vi "WS_BackCheck_Serial.vi"(2 "stationName":string, 3 "serialNumber":string) -> (0 "ProcessName":string, 1 "Status":i8)   [LabVIEW 2022 SP3]
uses:
  C:/Users/K90011729/OneDrive - Kimball Electronics/Desktop/Proyectos/IPB2 Test secuence/WsConnector/WSConnector.dll
  WSConnector.dll
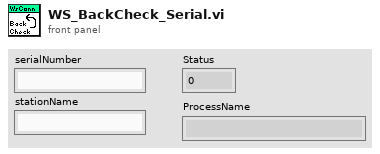
[diagram p1: front panel]
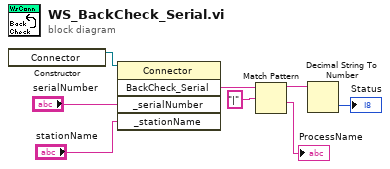
[diagram p0: block diagram]
diagram:
  n1 = constructor class="Connector"() -> (reference out=w8:refnum<k24>)  [unwired: 3 in, 2 out]
  n2 = invoke class="Connector" method="BackCheck_Serial"(reference=w8, "_serialNumber"="serialNumber", "_stationName"="stationName") -> ("BackCheck_Serial"=w2:string)  [unwired: 2 in, 4 out]
  n3 = Match Pattern(string=w2, regular expression="|") -> (before substring=w4:string, after substring=→"ProcessName":string)  [unwired: 1 in, 2 out]
  n4 = Decimal String To Number(string=w4) -> (number=→"Status":i32)  [unwired: 2 in, 1 out]
